vi "Bool to String.vi"(11 "Boolean":bool) -> (3 "Value":string)   [LabVIEW 2018, in "JSON.lvlib"]
uses:
  JSON.lvlib
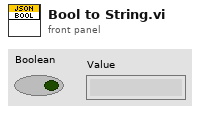
[diagram p1: front panel]
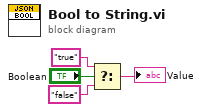
[diagram p0: block diagram]
diagram:
  n1 = Select(t="true", s="Boolean", f="false") -> (s? t:f=→"Value":string)
